vi "Actor Core.vi"(8 "error in":errorcluster, 11 "subpanel 1 in":refnum<class "subpanel 1.lvclass">) -> (0 "error out":errorcluster, 3 "Actor out":refnum<class "Actor.lvclass">)   [LabVIEW 2023, in "subpanel 1.lvclass"]
doc: "(<B>Filename</B>: Actor Framework.lvlib:Actor.lvclass:Actor Core.vi)\n\nReceives messages to the actor, reacts to them, and initiates any error handling that may shut the actor down.\n\nDescendant classes may override this VI to append parallel tasks for the actor to complete while it handles messages. Overrides use the Call Parent Method node."
uses:
  subpanel 1.lvclass
  <vilib>/ActorFramework/Actor/Actor.lvclass
  subpanel/subpanel (abstract).lvclass
  N:/VT LTT Project/Source Code/GUI/Reused Code/Subpanels Actor/subpanels/subpanel/subpanel (abstract).lvclass
  C:/Program Files/National Instruments/LabVIEW 2023/vi.lib/ActorFramework/Actor/Actor.lvclass
  N:/VT LTT Project/Source Code/GUI/Reused Code/Subpanels Actor/subpanels/subpanel 1/subpanel 1.lvclass
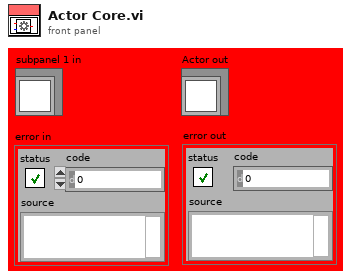
[diagram p1: front panel]
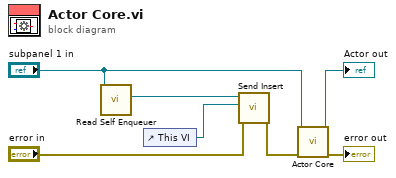
[diagram p0: block diagram]
diagram:
  n1 = call <vilib>:"Read Self Enqueuer.vi"("Actor"="subpanel 1 in") -> ("Self Enqueuer"=w4:refnum<class "Message Enqueuer.lvclass">)  [unwired: 10 in]
  n2 = control-ref of="This VI"() -> (w1:refnum<vi>)
  n3 = call "Send Insert.vi"("error in (no error)"="error in", "VI Ref"=w1, "Message Enqueuer"=w4) -> ("error out"=w2:errorcluster)  [unwired: 7 in, 1 out]
  n4 = call-parent "Actor Core.vi"("error in"=w2, "Actor in"="subpanel 1 in") -> ("error out"=→"error out":errorcluster, "Actor out"=→"Actor out":refnum<class "Actor.lvclass">)  [unwired: 8 in]
